vi "Normalize Quaternion.vi"(1 "quaternion":T1) -> (0 "normalized quaternion":dbl)   [LabVIEW 2017, in "NI_Kinematics.lvlib"]
doc: "Returns the norm of the input <B>quaternion</B>. This VI uses the Vector Norm VI to compute the norm. \n\n<B>.m file:</B> norm"
uses:
  <vilib>/robotics/Kinematics/NI_Kinematics.lvlib
  <vilib>/robotics/Kinematics/Quaternion.ctl
  <vilib>/Analysis/_algsub.llb/Real Vector Norm.vi
  <vilib>/Analysis/NI_AALPro.lvlib
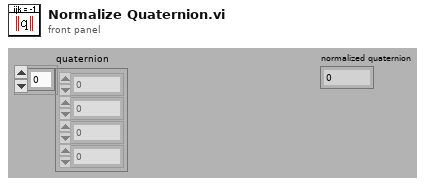
[diagram p1: front panel]
types:
  T1 = typedef "NI_Kinematics.lvlib/Quaternion.ctl" = dbl[]
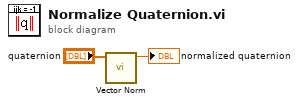
[diagram p0: block diagram]
diagram:
  n1 = call-poly <vilib>:"Vector Norm.vi"("Input Vector"="quaternion") -> ("norm"=→"normalized quaternion":dbl)  [unwired: 2 in, 8 out]
